vi "Global_CMD_SEN_Data In.vi"() -> ()   [LabVIEW 2020, in "Swerve_Odometry_SEN.lvlib"]
uses:
  startup.rtexe/Swerve_Odometry_SEN.lvlib
panel:
  in  "Tracking":bool=TRUE
  in  "Offset Values":cluster{"Y":dbl, "X":dbl, "Degrees":dbl}
  # "The Names of the Data items in the Global Variable MUST describe who the Single Writer is\nFor Command Globals the Commander(CMD) represents Teleop or Autonomous or other command loop.\nThe naming convention for a Command Sensor Global is:   \n\nCMD_SEN_SubSystem_Data Name\n\nExample:\nCMD_SEN_Gyro_Reset\nCMD_SEN_Distance_SetZero"
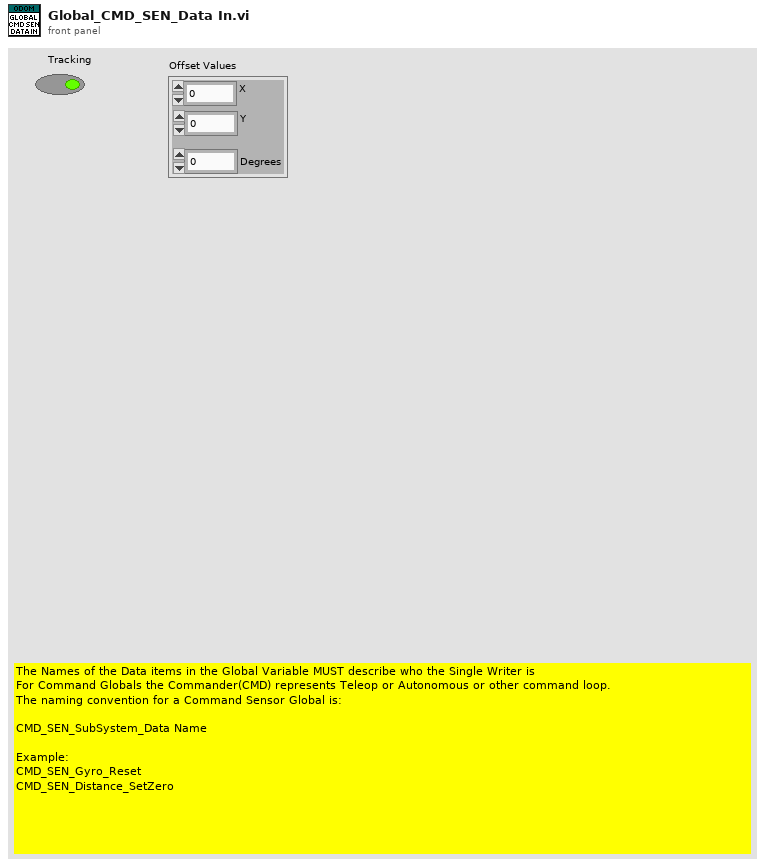
[diagram p1: front panel]
diagram:
